vi "FCET_Action_ReadExcelSettings_Sub.vi"(4 "TDefPath":path, 6 "WriteEnums":bool, 7 "Start_Cell":string, 8 "error in":errorcluster, 9 "Sheet":string, 11 "Data":string[][](array[string])) -> (0 "error out":errorcluster)   [LabVIEW 2017]
uses:
  FCET_Globals_V001.llb/Globals_Settings_FCE_TS.vi
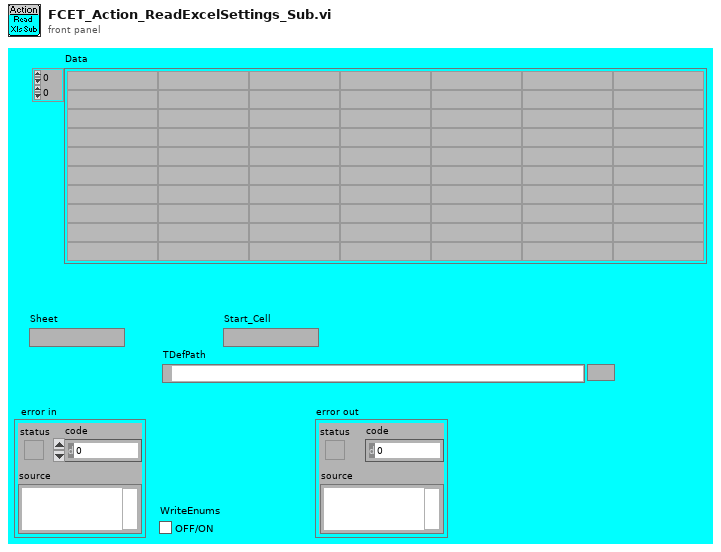
[diagram p1: front panel]
types:
  T1 = enum16{"Volts", "Amps", "Deg F", "Deg C", "Deg R", "Kelvins", "Strain", "Ohms", "Hz", "Seconds", "Meters", "Inches", "Degrees", "Radians", "g", "m/s^2", "Pascals", "From TEDS"}
  T2 = typedef "FCE_TS_EIP_TypeDefs_Cluster AI.ctl" = cluster{"Ena":bool[], "Signal Name":string[], "Description":string[], "Phys Unit":string[], "SensorType":enum16{"Voltage", "Current", "PT1000"}[], "ModAdd":u16[], "Chan":u16[], "Raw Min":sgl[], "Raw Max":sgl[], "Phys Min":sgl[], "Phys Max":sgl[], "Offset":sgl[], "Raw Unit":enum16{"Volts", "mAmps", "°C"}[]}
  T3 = typedef "FCE_TS_EIP_TypeDefs_Cluster_AO.ctl" = cluster{"Ena":bool[], "Signal Name":string[], "Description":string[], "Phys Unit":string[], "SensorType":enum16{"Voltage", "Current"}[], "ModAdd":u16[], "Chan":u16[], "Raw Min":sgl[], "Raw Max":sgl[], "Phys Min":sgl[], "Phys Max":sgl[], "Default":sgl[], "Raw Unit":enum16{"Volts", "Amps", "Deg F", "Deg C", "Deg R", "Kelvins", "Strain", "Ohms", "Hz", "Seconds", "Meters", "Inches", "Degrees", "Radians", "g", "m/s^2", "Pascals", "From TEDS"}[]}
  T4 = cluster{"Name":string[], "Index":i32[], "Ena":u32[], "Limits I":sgl[][], "Delays_I":i32[][], "Limits II":sgl[][], "Delays_II":i32[][], "Limits_III":sgl[][], "Delays_III":i32[][], "Message":string[]}
  T5 = cluster{"Name":string[], "Index":i32[], "Ena":u32[], "Alarm_Cond":bool[], "I":bool[], "Delay_I":i32[], "II":bool[], "Delay_II":i32[], "III":bool[], "Delay_III":i32[], "Message":string[]}
  T6 = typedef "FCE_TS_EIP_TypeDefs_Cluster DI.ctl" = cluster{"Signal Name":string[], "Description":string[], "Port":u16[], "Chan":u16[], "Inv":bool[], "Addr":u16[]}
  T7 = typedef "FCE_TS_EIP_TypeDefs_Cluster DO.ctl" = cluster{"Def":bool[], "Signal Name":string[], "Description":string[], "Port":u16[], "Chan":u16[], "Inv":bool[], "Addr":u16[]}
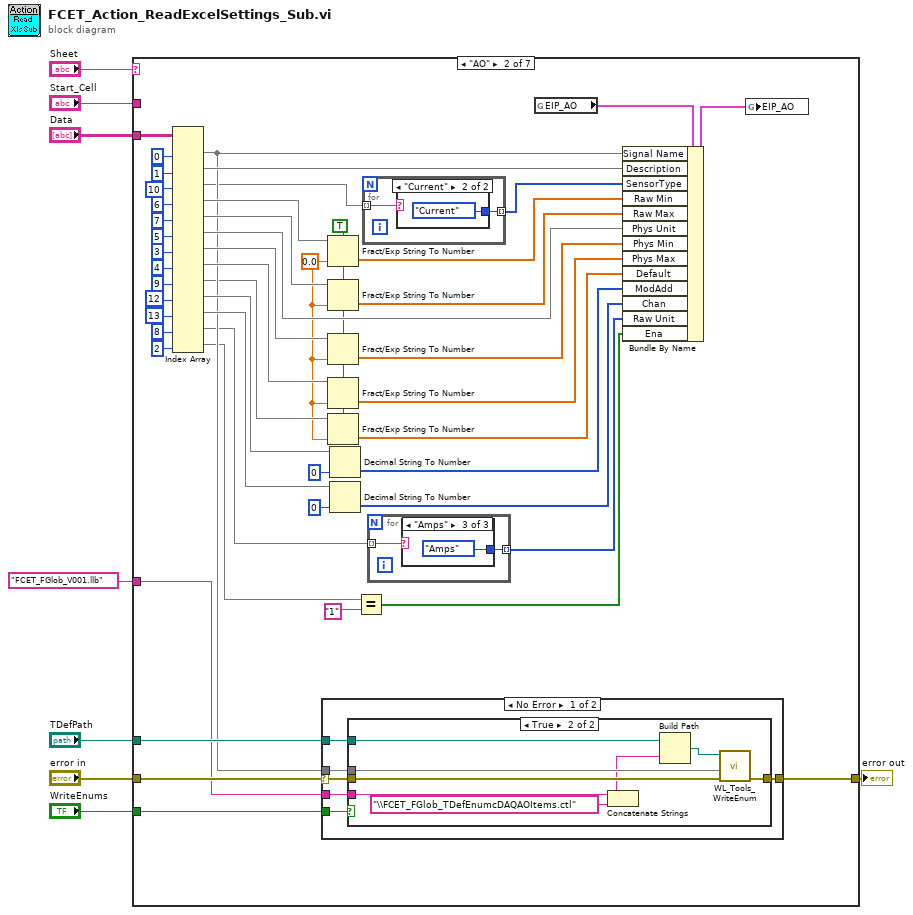
[diagram p0: block diagram]
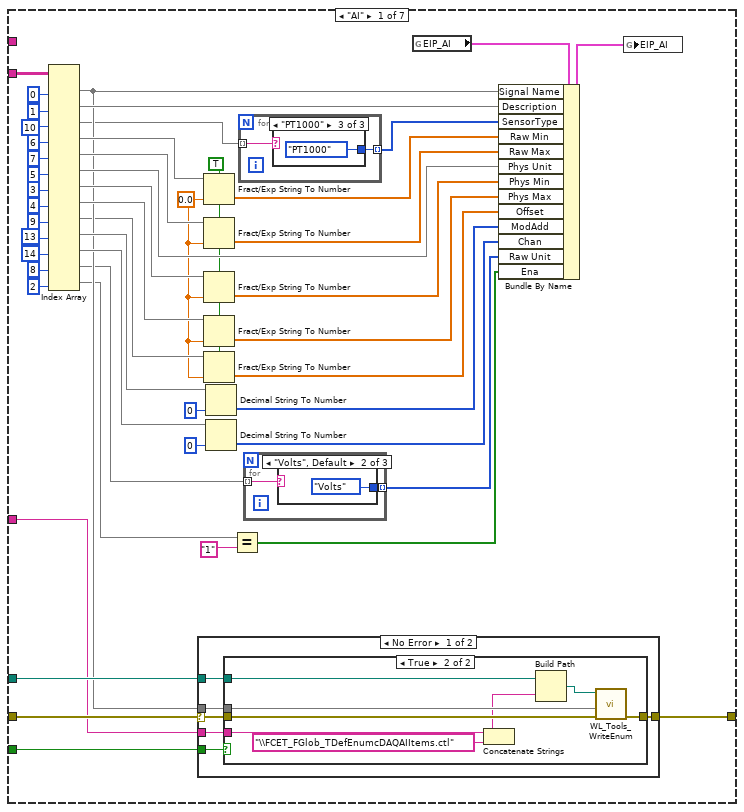
[diagram p2: hidden frame]
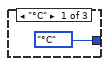
[diagram p3: hidden frame]
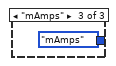
[diagram p4: hidden frame]
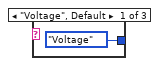
[diagram p5: hidden frame]
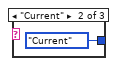
[diagram p6: hidden frame]
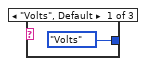
[diagram p9: hidden frame]
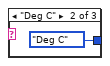
[diagram p10: hidden frame]
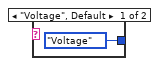
[diagram p11: hidden frame]
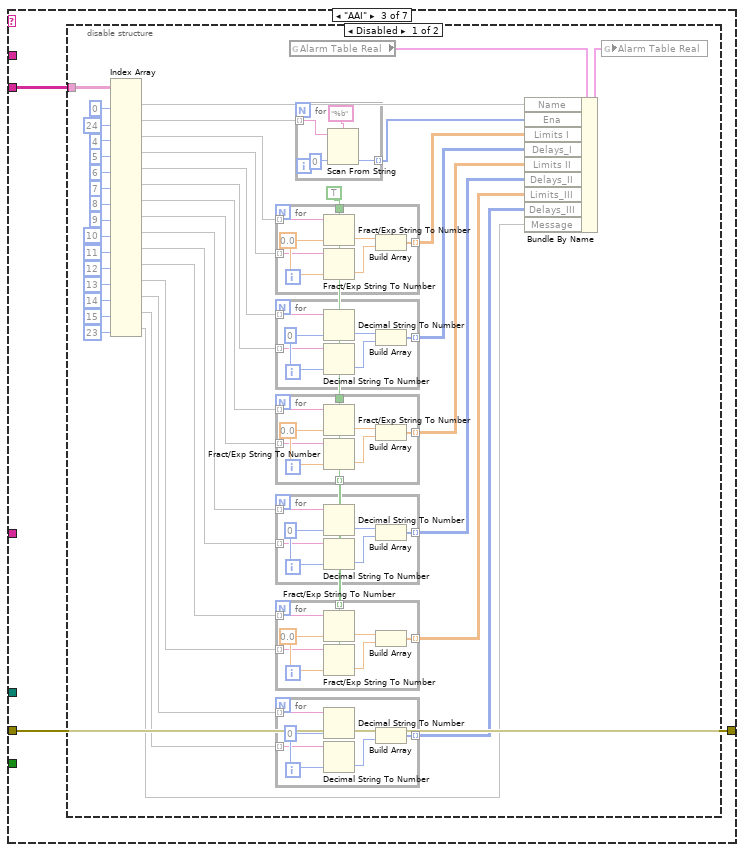
[diagram p14: hidden frame]
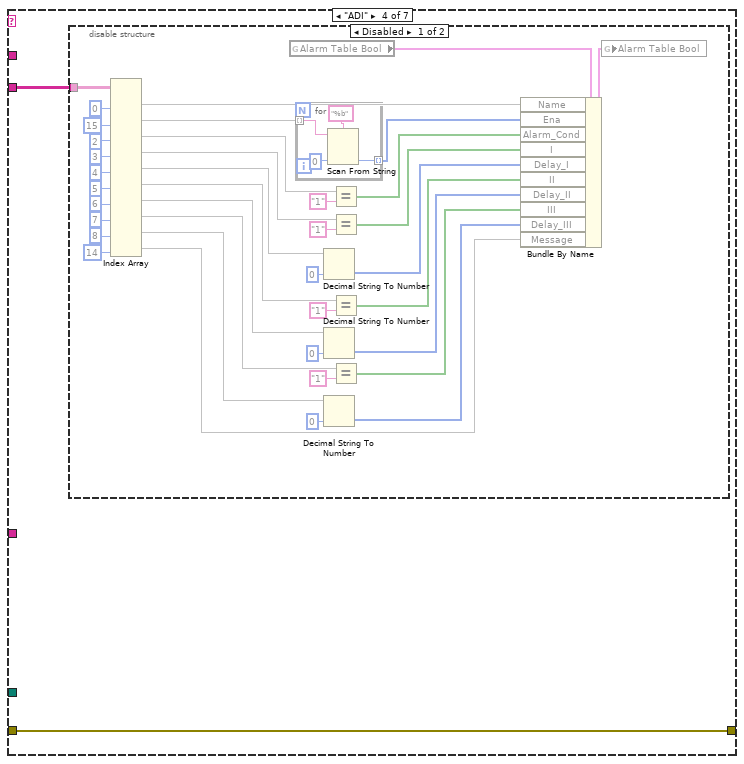
[diagram p16: hidden frame]
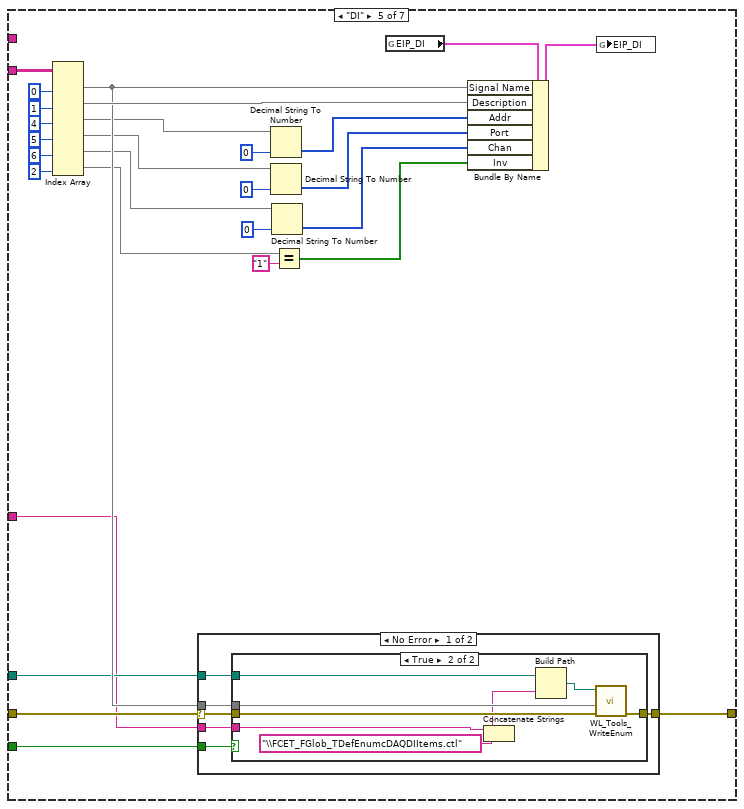
[diagram p18: hidden frame]
diagram:
  n1 = case shown="\"AO\"" "Sheet" {
    tunnel: "Data" -> [w57 w132 w159 w246 w316 w364 _]
    tunnel: "error in" -> [w37 w112 w158 w245 w312 w360 w381]
    tunnel: "WriteEnums" -> [w36 w111 _ _ w311 w359 _]
    tunnel: [w35 w110 w158 w245 w309 w357 w381] -> w4
    tunnel: "TDefPath" -> [w34 w109 _ _ w308 w356 _]
    tunnel: "Start_Cell" -> [_ _ _ _ _ _ _]
    tunnel: "FCET_FGlob_V001.llb" ("string") -> [w29 w104 _ _ w302 w350 _]
    frame "AI" {
      w18 = sgl 0.0 ("default (0 DBL)")
      w17 = TRUE ("use system decimal point (T)")
      n2 = Index Array(array=w57, index (col) #1=0 ("disabled index (col)"), index (col) #2=1 ("disabled index (col)"), index (col) #3=10 ("disabled index (col)"), index (col) #4=6 ("disabled index (col)"), index (col) #5=7 ("disabled index (col)"), index (col) #6=5 ("disabled index (col)"), index (col) #7=3 ("disabled index (col)"), index (col) #8=4 ("disabled index (col)"), index (col) #9=9 ("disabled index (col)"), index (col) #10=13 ("disabled index (col)"), index (col) #11=14 ("disabled index (col)"), index (col) #12=8 ("disabled index (col)"), index (col) #13=2 ("index (col)")) -> (element #1=w22:string[], element #2=w54:string[], element #3=w21:string[], element #4=w51:string[], element #5=w47:string[], element #6=w45:string[], element #7=w41:string[], element #8=w40:string[], element #9=w19:string[], element #10=w32:string[], element #11=w26:string[], element #12=w14:string[], element #13=w12:string[])  [unwired: 13 in]
      n3 = case shown="No Error" w37 {
        selector: w37 -> [w71 w83]
        tunnel: w36 -> [w72 _]
        tunnel: w22 -> [w73 _]
        tunnel: [w70 w83] -> w35
        tunnel: w34 -> [w69 _]
        tunnel: w29 -> [w68 _]
        frame No Error {
          n4 = case shown="True" w72 {
            tunnel: w73 -> [_ w80]
            tunnel: w71 -> [w74 w82]
            tunnel: [w74 w81] -> w70
            tunnel: w69 -> [_ w79]
            tunnel: w68 -> [_ w75]
            frame False {
            }
            frame True {
              n5 = Concatenate Strings(w75, "\\FCET_FGlob_TDefEnumcDAQAIItems.ctl" ("string")) -> (w76:string)
              n6 = Build Path(base path=w79, name or relative path=w76) -> (appended path=w78:path)
              n7 = call "WL_Tools_WriteEnum.vi"("err in"=w82, "Strings"=w80, "BasePath"=w78) -> ("err out"=w81:errorcluster)  [unwired: 8 in]
            }
          }
        }
        frame Error {
        }
      }
      n8 = Fract/Exp String To Number(use system decimal point (T)=w17, string=w51, default (0 dbl)=w18) -> (number=w50:sgl[])  [unwired: 1 in, 1 out]
      n9 = Fract/Exp String To Number(use system decimal point (T)=w17, string=w47, default (0 dbl)=w18) -> (number=w48:sgl[])  [unwired: 1 in, 1 out]
      n10 = Fract/Exp String To Number(use system decimal point (T)=w17, string=w41, default (0 dbl)=w18) -> (number=w38:sgl[])  [unwired: 1 in, 1 out]
      n11 = Fract/Exp String To Number(use system decimal point (T)=w17, string=w40, default (0 dbl)=w18) -> (number=w39:sgl[])  [unwired: 1 in, 1 out]
      n12 = Fract/Exp String To Number(use system decimal point (T)=w17, string=w19, default (0 dbl)=w18) -> (number=w16:sgl[])  [unwired: 1 in, 1 out]
      n13 = Decimal String To Number(string=w32, default (0L)=u16 0 ("default (0 U32)")) -> (number=w30:u16[])  [unwired: 1 in, 1 out]
      n14 = Decimal String To Number(string=w26, default (0L)=u16 0 ("default (0 U32)")) -> (number=w25:u16[])  [unwired: 1 in, 1 out]
      n15 = Equal?(x=w12, y="1" ("String")) -> (x = y?=w9:bool[])
      n16 = for {
        tunnel: w21 -> [w64] mode=indexing
        tunnel: [w63] -> w20 mode=indexing
        n17 = case shown="\"PT1000\"" w64 {
          tunnel: [enum16{"Voltage", "Current", "PT1000"}."Voltage" ("Analog Input") enum16{"Voltage", "Current", "PT1000"}."Current" ("Analog Input") enum16{"Voltage", "Current", "PT1000"}."PT1000" ("Analog Input")] -> w63
          frame "Voltage", Default {
          }
          frame "Current" {
          }
          frame "PT1000" {
          }
        }
      }
      n18 = for {
        tunnel: w14 -> [w59] mode=indexing
        tunnel: [w58] -> w15 mode=indexing
        n19 = case shown="\"Volts\", Default" w59 {
          tunnel: [enum16{"Volts", "mAmps", "°C"}."°C" ("RawUnit") enum16{"Volts", "mAmps", "°C"}."Volts" ("RawUnit") enum16{"Volts", "mAmps", "°C"}."mAmps" ("RawUnit")] -> w58
          frame "°C" {
          }
          frame "Volts", Default {
          }
          frame "mAmps" {
          }
        }
      }
      n20 = global read "Globals_Settings_FCE_TS.vi" "EIP_AI"() -> (w24:T2)
      n21 = Bundle By Name(cluster=w24, "Signal Name"=w22, "Description"=w54, "SensorType"=w20, "Raw Min"=w50, "Raw Max"=w48, "Phys Unit"=w45, "Phys Min"=w38, "Phys Max"=w39, "Offset"=w16, "ModAdd"=w30, "Chan"=w25, "Raw Unit"=w15, "Ena"=w9) -> (w23:T2)
      n22 = global write "Globals_Settings_FCE_TS.vi" "EIP_AI"(w23) -> ()
    }
    frame "AO" {
      w93 = sgl 0.0 ("default (0 DBL)")
      w92 = TRUE ("use system decimal point (T)")
      n23 = Index Array(array=w132, index (col) #1=0 ("disabled index (col)"), index (col) #2=1 ("disabled index (col)"), index (col) #3=10 ("disabled index (col)"), index (col) #4=6 ("disabled index (col)"), index (col) #5=7 ("disabled index (col)"), index (col) #6=5 ("disabled index (col)"), index (col) #7=3 ("disabled index (col)"), index (col) #8=4 ("disabled index (col)"), index (col) #9=9 ("disabled index (col)"), index (col) #10=12 ("disabled index (col)"), index (col) #11=13 ("disabled index (col)"), index (col) #12=8 ("disabled index (col)"), index (col) #13=2 ("index (col)")) -> (element #1=w97:string[], element #2=w129:string[], element #3=w96:string[], element #4=w126:string[], element #5=w122:string[], element #6=w120:string[], element #7=w116:string[], element #8=w115:string[], element #9=w94:string[], element #10=w107:string[], element #11=w101:string[], element #12=w89:string[], element #13=w87:string[])  [unwired: 13 in]
      n24 = case shown="No Error" w112 {
        selector: w112 -> [w145 w157]
        tunnel: w111 -> [w146 _]
        tunnel: w97 -> [w147 _]
        tunnel: [w144 w157] -> w110
        tunnel: w109 -> [w143 _]
        tunnel: w104 -> [w142 _]
        frame No Error {
          n25 = case shown="True" w146 {
            tunnel: w147 -> [_ w154]
            tunnel: w145 -> [w148 w156]
            tunnel: [w148 w155] -> w144
            tunnel: w143 -> [_ w153]
            tunnel: w142 -> [_ w149]
            frame False {
            }
            frame True {
              n26 = Concatenate Strings(w149, "\\FCET_FGlob_TDefEnumcDAQAOItems.ctl" ("string")) -> (w150:string)
              n27 = Build Path(base path=w153, name or relative path=w150) -> (appended path=w152:path)
              n28 = call "WL_Tools_WriteEnum.vi"("err in"=w156, "Strings"=w154, "BasePath"=w152) -> ("err out"=w155:errorcluster)  [unwired: 8 in]
            }
          }
        }
        frame Error {
        }
      }
      n29 = Fract/Exp String To Number(use system decimal point (T)=w92, string=w126, default (0 dbl)=w93) -> (number=w125:sgl[])  [unwired: 1 in, 1 out]
      n30 = Fract/Exp String To Number(use system decimal point (T)=w92, string=w122, default (0 dbl)=w93) -> (number=w123:sgl[])  [unwired: 1 in, 1 out]
      n31 = Fract/Exp String To Number(use system decimal point (T)=w92, string=w116, default (0 dbl)=w93) -> (number=w113:sgl[])  [unwired: 1 in, 1 out]
      n32 = Fract/Exp String To Number(use system decimal point (T)=w92, string=w115, default (0 dbl)=w93) -> (number=w114:sgl[])  [unwired: 1 in, 1 out]
      n33 = Fract/Exp String To Number(use system decimal point (T)=w92, string=w94, default (0 dbl)=w93) -> (number=w91:sgl[])  [unwired: 1 in, 1 out]
      n34 = Decimal String To Number(string=w107, default (0L)=u16 0 ("default (0 U32)")) -> (number=w105:u16[])  [unwired: 1 in, 1 out]
      n35 = Decimal String To Number(string=w101, default (0L)=u16 0 ("default (0 U32)")) -> (number=w100:u16[])  [unwired: 1 in, 1 out]
      n36 = Equal?(x=w87, y="1" ("String")) -> (x = y?=w84:bool[])
      n37 = for {
        tunnel: w96 -> [w139] mode=indexing
        tunnel: [w138] -> w95 mode=indexing
        n38 = case shown="\"Current\"" w139 {
          tunnel: [enum16{"Voltage", "Current"}."Voltage" ("Analog Input") enum16{"Voltage", "Current"}."Current" ("Analog Input")] -> w138
          frame "Voltage", Default {
          }
          frame "Current" {
          }
        }
      }
      n39 = for {
        tunnel: w89 -> [w134] mode=indexing
        tunnel: [w133] -> w90 mode=indexing
        n40 = case shown="\"Amps\"" w134 {
          tunnel: [T1."Volts" ("RawUnit") T1."Deg C" ("RawUnit") T1."Amps" ("RawUnit")] -> w133
          frame "Volts", Default {
          }
          frame "Deg C" {
          }
          frame "Amps" {
          }
        }
      }
      n41 = global read "Globals_Settings_FCE_TS.vi" "EIP_AO"() -> (w99:T3)
      n42 = Bundle By Name(cluster=w99, "Signal Name"=w97, "Description"=w129, "SensorType"=w95, "Raw Min"=w125, "Raw Max"=w123, "Phys Unit"=w120, "Phys Min"=w113, "Phys Max"=w114, "Default"=w91, "ModAdd"=w105, "Chan"=w100, "Raw Unit"=w90, "Ena"=w84) -> (w98:T3)
      n43 = global write "Globals_Settings_FCE_TS.vi" "EIP_AO"(w98) -> ()
    }
    frame "AAI" {
      n44 = disable-structure shown="Disabled" {
        disable-tunnel: w159 -> [w199 _]
        frame Disabled {
          w183 = TRUE ("use system decimal point (T)")
          n45 = Index Array(array=w199, index (col) #1=0 ("disabled index (col)"), index (col) #2=24 ("disabled index (col)"), index (col) #3=4 ("disabled index (col)"), index (col) #4=5 ("disabled index (col)"), index (col) #5=6 ("disabled index (col)"), index (col) #6=7 ("disabled index (col)"), index (col) #7=8 ("disabled index (col)"), index (col) #8=9 ("disabled index (col)"), index (col) #9=10 ("disabled index (col)"), index (col) #10=11 ("disabled index (col)"), index (col) #11=12 ("disabled index (col)"), index (col) #12=13 ("disabled index (col)"), index (col) #13=14 ("disabled index (col)"), index (col) #14=15 ("disabled index (col)"), index (col) #15=23 ("disabled index (col)")) -> (element #1=w189:string[], element #2=w188:string[], element #3=w186:string[], element #4=w185:string[], element #5=w182:string[], element #6=w181:string[], element #7=w179:string[], element #8=w178:string[], element #9=w174:string[], element #10=w173:string[], element #11=w169:string[], element #12=w168:string[], element #13=w164:string[], element #14=w163:string[], element #15=w160:string[])  [unwired: 15 in]
          n46 = for {
            tunnel: w183 -> [w239]
            tunnel: w186 -> [w238] mode=indexing
            tunnel: w185 -> [w237] mode=indexing
            tunnel: [w234] -> w184 mode=indexing
            w240 = sgl 0.0 ("default (0 DBL)")
            n47 = Fract/Exp String To Number(use system decimal point (T)=w239, string=w238, default (0 dbl)=w240) -> (number=w236:sgl)  [unwired: 1 in, 1 out]
            n48 = Fract/Exp String To Number(use system decimal point (T)=w239, string=w237, default (0 dbl)=w240) -> (number=w235:sgl)  [unwired: 1 in, 1 out]
            n49 = Build Array(w236, w235) -> (w234:sgl[])
          }
          n50 = for {
            tunnel: w181 -> [w225] mode=indexing
            tunnel: [w222] -> w180 mode=indexing
            tunnel: w182 -> [w221] mode=indexing
            w226 = 0 ("default (0 DBL)")
            n51 = Decimal String To Number(string=w221, default (0L)=w226) -> (number=w224:i32)  [unwired: 1 in, 1 out]
            n52 = Decimal String To Number(string=w225, default (0L)=w226) -> (number=w223:i32)  [unwired: 1 in, 1 out]
            n53 = Build Array(w224, w223) -> (w222:i32[])
          }
          n54 = for {
            tunnel: w183 -> [w227]
            tunnel: w179 -> [w232] mode=indexing
            tunnel: w178 -> [w231] mode=indexing
            tunnel: [w228] -> w177 mode=indexing
            tunnel: [w227] -> w171 mode=indexing
            w233 = sgl 0.0 ("default (0 DBL)")
            n55 = Fract/Exp String To Number(use system decimal point (T)=w227, string=w232, default (0 dbl)=w233) -> (number=w230:sgl)  [unwired: 1 in, 1 out]
            n56 = Fract/Exp String To Number(use system decimal point (T)=w227, string=w231, default (0 dbl)=w233) -> (number=w229:sgl)  [unwired: 1 in, 1 out]
            n57 = Build Array(w230, w229) -> (w228:sgl[])
          }
          n58 = for {
            tunnel: w173 -> [w219] mode=indexing
            tunnel: [w216] -> w172 mode=indexing
            tunnel: w174 -> [w215] mode=indexing
            w220 = 0 ("default (0 DBL)")
            n59 = Decimal String To Number(string=w215, default (0L)=w220) -> (number=w218:i32)  [unwired: 1 in, 1 out]
            n60 = Decimal String To Number(string=w219, default (0L)=w220) -> (number=w217:i32)  [unwired: 1 in, 1 out]
            n61 = Build Array(w218, w217) -> (w216:i32[])
          }
          n62 = for {
            tunnel: w171 -> [w213] mode=indexing
            tunnel: w169 -> [w212] mode=indexing
            tunnel: w168 -> [w211] mode=indexing
            tunnel: [w208] -> w167 mode=indexing
            w214 = sgl 0.0 ("default (0 DBL)")
            n63 = Fract/Exp String To Number(use system decimal point (T)=w213, string=w212, default (0 dbl)=w214) -> (number=w210:sgl)  [unwired: 1 in, 1 out]
            n64 = Fract/Exp String To Number(use system decimal point (T)=w213, string=w211, default (0 dbl)=w214) -> (number=w209:sgl)  [unwired: 1 in, 1 out]
            n65 = Build Array(w210, w209) -> (w208:sgl[])
          }
          n66 = for {
            tunnel: w163 -> [w206] mode=indexing
            tunnel: [w203] -> w162 mode=indexing
            tunnel: w164 -> [w202] mode=indexing
            w207 = 0 ("default (0 DBL)")
            n67 = Decimal String To Number(string=w202, default (0L)=w207) -> (number=w205:i32)  [unwired: 1 in, 1 out]
            n68 = Decimal String To Number(string=w206, default (0L)=w207) -> (number=w204:i32)  [unwired: 1 in, 1 out]
            n69 = Build Array(w205, w204) -> (w203:i32[])
          }
          n70 = global read "Globals_Settings_FCE_TS.vi" "Alarm Table Real"() -> (w201:T4)
          n71 = for {
            tunnel: w188 -> [w242] mode=indexing
            tunnel: [w241] -> w187 mode=indexing
            n72 = Scan From String(format string="%b", input string=w242, default 1=u32 0) -> (output 1=w241:u32)  [unwired: 2 in, 3 out]
          }
          n73 = Bundle By Name(cluster=w201, "Name"=w189, "Ena"=w187, "Limits I"=w184, "Delays_I"=w180, "Limits II"=w177, "Delays_II"=w172, "Limits_III"=w167, "Delays_III"=w162, "Message"=w160) -> (w200:T4)
          n74 = global write "Globals_Settings_FCE_TS.vi" "Alarm Table Real"(w200) -> ()
        }
        frame Enabled {
        }
      }
    }
    frame "ADI" {
      n75 = disable-structure shown="Disabled" {
        disable-tunnel: w246 -> [w282 _]
        frame Disabled {
          n76 = Index Array(array=w282, index (col) #1=0 ("disabled index (col)"), index (col) #2=15 ("disabled index (col)"), index (col) #3=2 ("disabled index (col)"), index (col) #4=3 ("disabled index (col)"), index (col) #5=4 ("disabled index (col)"), index (col) #6=5 ("disabled index (col)"), index (col) #7=6 ("disabled index (col)"), index (col) #8=7 ("disabled index (col)"), index (col) #9=8 ("disabled index (col)"), index (col) #10=14 ("disabled index (col)")) -> (element #1=w272:string[], element #2=w271:string[], element #3=w268:string[], element #4=w265:string[], element #5=w262:string[], element #6=w259:string[], element #7=w256:string[], element #8=w253:string[], element #9=w247:string[], element #10=w249:string[])  [unwired: 10 in]
          n77 = global read "Globals_Settings_FCE_TS.vi" "Alarm Table Bool"() -> (w284:T5)
          n78 = for {
            tunnel: w271 -> [w286] mode=indexing
            tunnel: [w285] -> w270 mode=indexing
            n79 = Scan From String(format string="%b", input string=w286, default 1=u32 0) -> (output 1=w285:u32)  [unwired: 2 in, 3 out]
          }
          n80 = Decimal String To Number(string=w262, default (0L)=0 ("default (0 DBL)")) -> (number=w261:i32[])  [unwired: 1 in, 1 out]
          n81 = Decimal String To Number(string=w256, default (0L)=0 ("default (0 DBL)")) -> (number=w255:i32[])  [unwired: 1 in, 1 out]
          n82 = Decimal String To Number(string=w247, default (0L)=0 ("default (0 DBL)")) -> (number=w250:i32[])  [unwired: 1 in, 1 out]
          n83 = Equal?(x=w268, y="1" ("String")) -> (x = y?=w267:bool[])
          n84 = Equal?(x=w265, y="1" ("String")) -> (x = y?=w264:bool[])
          n85 = Equal?(x=w259, y="1" ("String")) -> (x = y?=w258:bool[])
          n86 = Equal?(x=w253, y="1" ("String")) -> (x = y?=w252:bool[])
          n87 = Bundle By Name(cluster=w284, "Name"=w272, "Ena"=w270, "Alarm_Cond"=w267, "I"=w264, "Delay_I"=w261, "II"=w258, "Delay_II"=w255, "III"=w252, "Delay_III"=w250, "Message"=w249) -> (w283:T5)
          n88 = global write "Globals_Settings_FCE_TS.vi" "Alarm Table Bool"(w283) -> ()
        }
        frame Enabled {
        }
      }
    }
    frame "DI" {
      n89 = Index Array(array=w316, index (col) #1=0 ("disabled index (col)"), index (col) #2=1 ("disabled index (col)"), index (col) #3=4 ("index (col)"), index (col) #4=5 ("index (col)"), index (col) #5=6 ("index (col)"), index (col) #6=2 ("index (col)")) -> (element #1=w310:string[], element #2=w313:string[], element #3=w292:string[], element #4=w303:string[], element #5=w289:string[], element #6=w291:string[])  [unwired: 6 in]
      n90 = case shown="No Error" w312 {
        selector: w312 -> [w320 w332]
        tunnel: w311 -> [w321 _]
        tunnel: w310 -> [w322 _]
        tunnel: [w319 w332] -> w309
        tunnel: w308 -> [w318 _]
        tunnel: w302 -> [w317 _]
        frame No Error {
          n91 = case shown="True" w321 {
            tunnel: w322 -> [_ w329]
            tunnel: w320 -> [w323 w331]
            tunnel: [w323 w330] -> w319
            tunnel: w318 -> [_ w328]
            tunnel: w317 -> [_ w324]
            frame False {
            }
            frame True {
              n92 = Concatenate Strings(w324, "\\FCET_FGlob_TDefEnumcDAQDIItems.ctl" ("string")) -> (w325:string)
              n93 = Build Path(base path=w328, name or relative path=w325) -> (appended path=w327:path)
              n94 = call "WL_Tools_WriteEnum.vi"("err in"=w331, "Strings"=w329, "BasePath"=w327) -> ("err out"=w330:errorcluster)  [unwired: 8 in]
            }
          }
        }
        frame Error {
        }
      }
      n95 = Decimal String To Number(string=w292, default (0L)=u16 0 ("default (0 U32)")) -> (number=w293:u16[])  [unwired: 1 in, 1 out]
      n96 = Decimal String To Number(string=w303, default (0L)=u16 0 ("default (0 U32)")) -> (number=w306:u16[])  [unwired: 1 in, 1 out]
      n97 = Decimal String To Number(string=w289, default (0L)=u16 0 ("default (0 U32)")) -> (number=w290:u16[])  [unwired: 1 in, 1 out]
      n98 = Equal?(x=w291, y="1") -> (x = y?=w296:bool[])
      n99 = global read "Globals_Settings_FCE_TS.vi" "EIP_DI"() -> (w299:T6)
      n100 = Bundle By Name(cluster=w299, "Signal Name"=w310, "Description"=w313, "Addr"=w293, "Port"=w306, "Chan"=w290, "Inv"=w296) -> (w298:T6)
      n101 = global write "Globals_Settings_FCE_TS.vi" "EIP_DI"(w298) -> ()
    }
    frame "DO" {
      n102 = Index Array(array=w364, index (col) #1=0 ("disabled index (col)"), index (col) #2=1 ("disabled index (col)"), index (col) #3=5 ("index (col)"), index (col) #4=6 ("index (col)"), index (col) #5=7 ("index (col)"), index (col) #6=2 ("index (col)"), index (col) #7=3 ("index (col)")) -> (element #1=w358:string[], element #2=w361:string[], element #3=w340:string[], element #4=w351:string[], element #5=w337:string[], element #6=w339:string[], element #7=w334:string[])  [unwired: 7 in]
      n103 = case shown="No Error" w360 {
        selector: w360 -> [w368 w380]
        tunnel: w359 -> [w369 _]
        tunnel: w358 -> [w370 _]
        tunnel: [w367 w380] -> w357
        tunnel: w356 -> [w366 _]
        tunnel: w350 -> [w365 _]
        frame No Error {
          n104 = case shown="True" w369 {
            tunnel: w370 -> [_ w377]
            tunnel: w368 -> [w371 w379]
            tunnel: [w371 w378] -> w367
            tunnel: w366 -> [_ w376]
            tunnel: w365 -> [_ w372]
            frame False {
            }
            frame True {
              n105 = Concatenate Strings(w372, "\\FCET_FGlob_TDefEnumcDAQDOItems.ctl" ("string")) -> (w373:string)
              n106 = Build Path(base path=w376, name or relative path=w373) -> (appended path=w375:path)
              n107 = call "WL_Tools_WriteEnum.vi"("err in"=w379, "Strings"=w377, "BasePath"=w375) -> ("err out"=w378:errorcluster)  [unwired: 8 in]
            }
          }
        }
        frame Error {
        }
      }
      n108 = Decimal String To Number(string=w340, default (0L)=u16 0 ("default (0 U32)")) -> (number=w341:u16[])  [unwired: 1 in, 1 out]
      n109 = Decimal String To Number(string=w351, default (0L)=u16 0 ("default (0 U32)")) -> (number=w354:u16[])  [unwired: 1 in, 1 out]
      n110 = Decimal String To Number(string=w337, default (0L)=u16 0 ("default (0 U32)")) -> (number=w338:u16[])  [unwired: 1 in, 1 out]
      n111 = Equal?(x=w339, y="1") -> (x = y?=w344:bool[])
      n112 = Equal?(x=w334, y="1") -> (x = y?=w333:bool[])
      n113 = global read "Globals_Settings_FCE_TS.vi" "EIP_DO"() -> (w347:T7)
      n114 = Bundle By Name(cluster=w347, "Signal Name"=w358, "Description"=w361, "Addr"=w341, "Port"=w354, "Chan"=w338, "Inv"=w344, "Def"=w333) -> (w346:T7)
      n115 = global write "Globals_Settings_FCE_TS.vi" "EIP_DO"(w346) -> ()
    }
    frame Default {
    }
  }
  "error out" <- w4
